vi "Command Wait.vi"(2 "Input Robot Commands":T1, 3 "Startup":bool, 4 "Cmd Parameter 4":string, 5 "Cmd Parameter 3":dbl, 6 "Cmd Parameter 2":dbl, 7 "Cmd Parameter 1":dbl) -> (0 "Output Robot Commands":T1, 1 "Completed":bool)   [LabVIEW 2016]
uses:
  Subsystems/All Robot Commands.ctl
  Subsystems/Drive and Climb SS/Drive + Climb Commands 2017.ctl
  Subsystems/Gear Delivery SS/Gear Delivery Commands.ctl
  Subsystems/Conveyor and Shooter SS/Conveyor and Shooter Commands.ctl
  Subsystems/Ball Intake SS/Ball Intake Commands.ctl
  Command Execution State.ctl
panel:
  # "Sample robot\ncontrol output.\nReplace with \nactual teleop \ncontrol signal \nstructure."
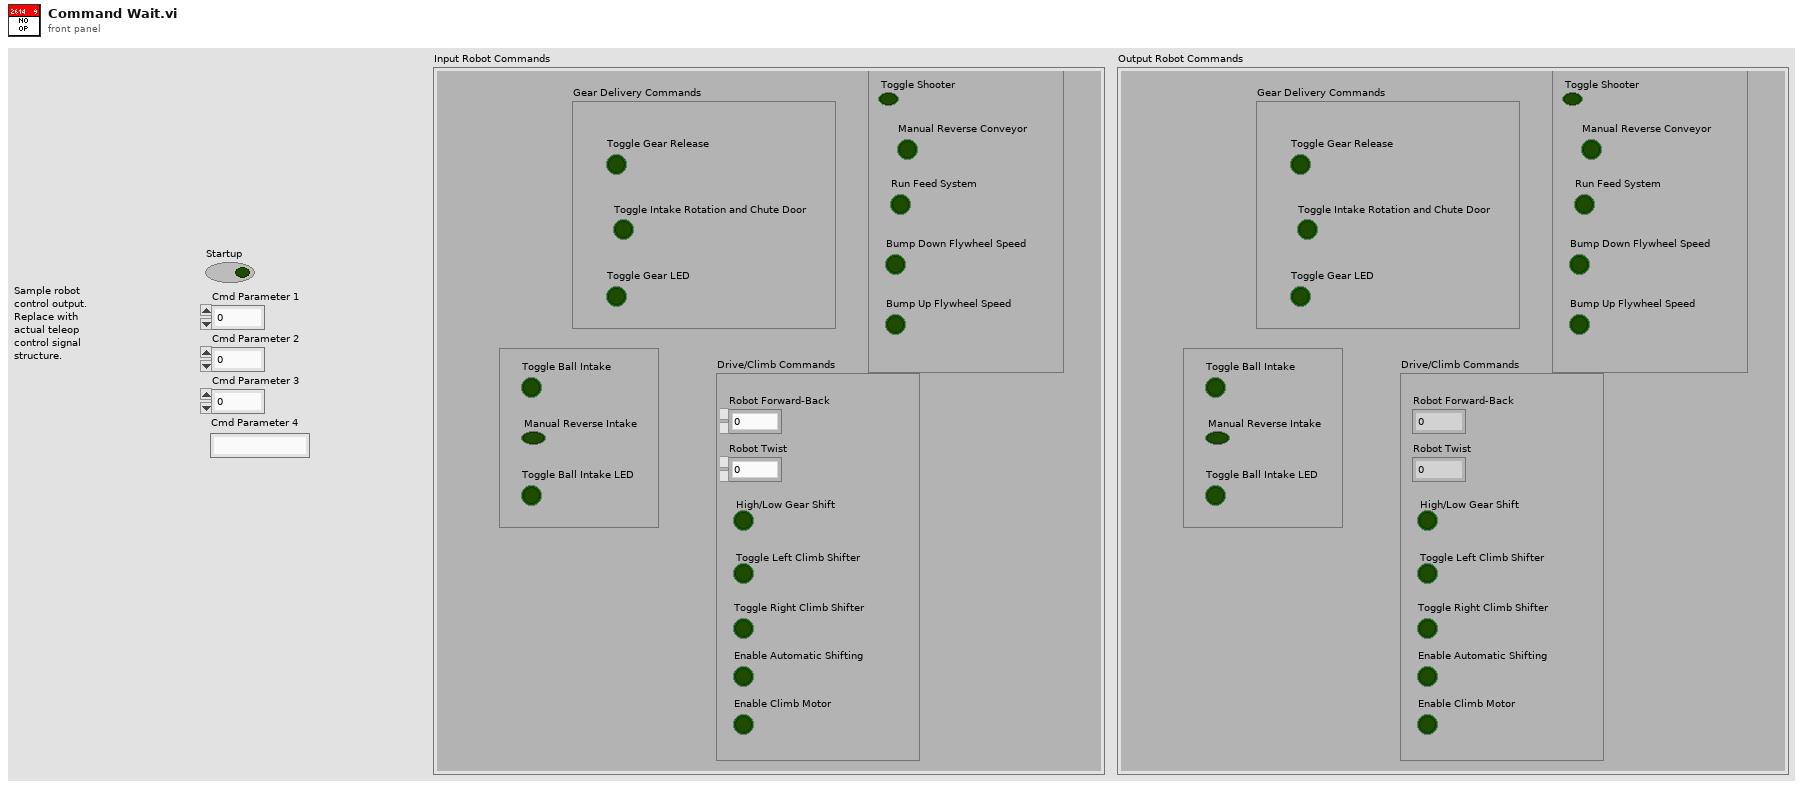
[diagram p1: front panel]
types:
  T1 = typedef "All Robot Commands.ctl" = cluster{"Drive/Climb Commands":T2, "Gear Delivery Commands":T3, "Shooter and Conveyor Commands":T4, "Ball Intake Commands":T5}
  T2 = typedef "Drive + Climb Commands 2017.ctl" = cluster{"Robot Forward-Back":dbl, "Robot Twist":dbl, "High/Low Gear Shift":bool, "Toggle Left Climb Shifter":bool, "Toggle Right Climb Shifter":bool, "Enable Automatic Shifting":bool, "Enable Climb Motor ":bool}
  T3 = typedef "Gear Delivery Commands.ctl" = cluster{"Toggle Gear Release":bool, "Toggle Intake Rotation and Chute Door":bool, "Toggle Gear LED":bool}
  T4 = typedef "Conveyor and Shooter Commands.ctl" = cluster{"Toggle Shooter":bool, "Manual Reverse Conveyor":bool, "Run Feed System":bool, "Bump Down Flywheel Speed":bool, "Bump Up Flywheel Speed":bool}
  T5 = typedef "Ball Intake Commands.ctl" = cluster{"Toggle Ball Intake":bool, "Manual Reverse Intake":bool, "Toggle Ball Intake LED":bool}
  T6 = typedef "Command Execution State.ctl" = enum16{"Initialize", "Execute", "Finish"}
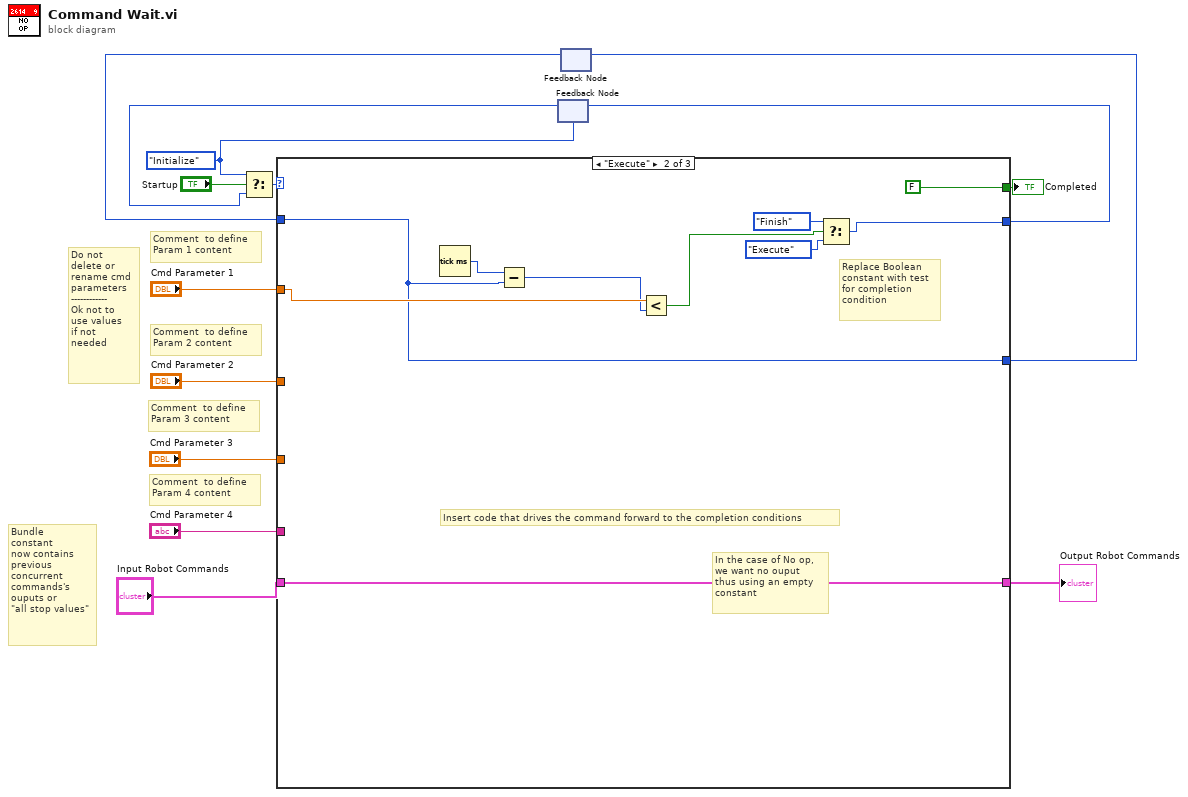
[diagram p0: block diagram]
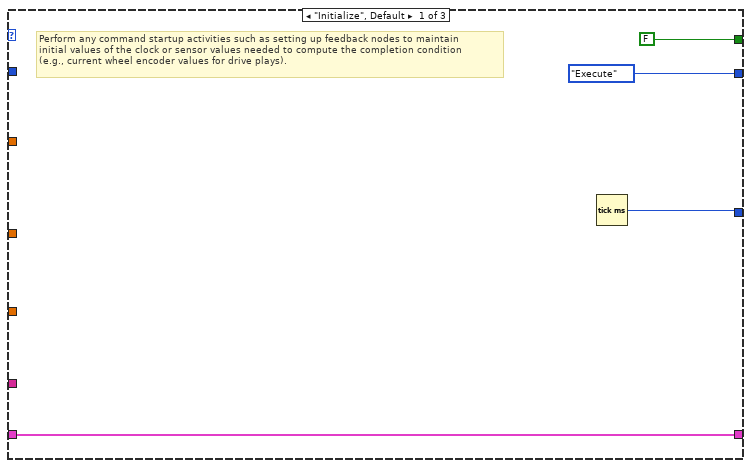
[diagram p2: hidden frame]
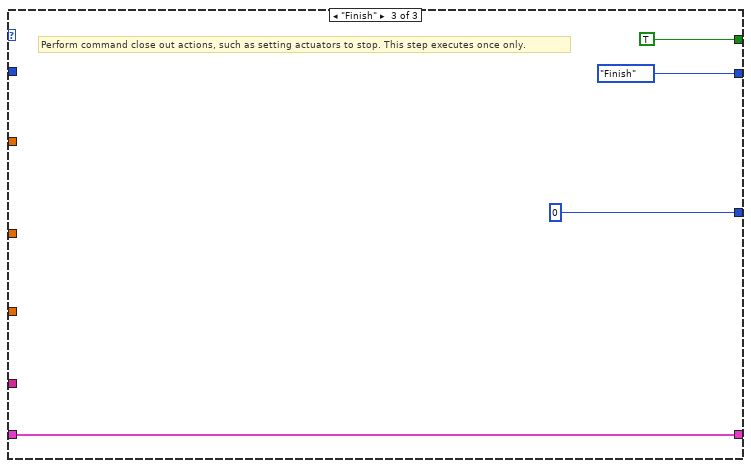
[diagram p3: hidden frame]
diagram:
  w9 = Command_Execution_State."Initialize" ("Play State")
  # "Comment  to define\nParam 4 content"
  # "Comment  to define\nParam 3 content"
  # "Bundle \nconstant\nnow contains\nprevious \nconcurrent\ncommands's\nouputs or\n\"all stop values\""
  # "Do not \ndelete or\nrename cmd\nparameters\n------------\nOk not to \nuse values\nif not \nneeded"
  # "Comment  to define\nParam 2 content"
  # "Comment  to define\nParam 1 content"
  n1 = feedback #1(w9) -> (w10:T6)
  n2 = Select(t=w9, s="Startup", f=w10) -> (s? t:f=w14:T6)
  n3 = feedback #2() -> (w1:u32)  [unwired: 1 in]
  n4 = case shown="\"Execute\"" w14 {
    tunnel: [FALSE FALSE TRUE] -> w12
    tunnel: [Command_Execution_State."Execute" ("Play State") w22 Command_Execution_State."Finish" ("f")] -> w11
    tunnel: "Cmd Parameter 1" -> [_ w26 _]
    tunnel: "Cmd Parameter 2" -> [_ _ _]
    tunnel: [w16 w27 w30] -> w5
    tunnel: "Input Robot Commands" -> [w16 w27 w30]
    tunnel: "Cmd Parameter 3" -> [_ _ _]
    tunnel: "Cmd Parameter 4" -> [_ _ _]
    tunnel: [w15 w19 0] -> w2
    tunnel: w1 -> [_ w19 _]
    frame "Initialize", Default {
      # "Perform any command startup activities such as setting up feedback nodes to maintain \ninitial values of the clock or sensor values needed to compute the completion condition\n(e.g., current wheel encoder values for drive plays)."
      n5 = Tick Count (ms)() -> (millisecond timer value=w15:u32)
    }
    frame "Execute" {
      # "In the case of No op, \nwe want no ouput \nthus using an empty \nconstant"
      # "Replace Boolean\nconstant with test \nfor completion \ncondition"
      # "Insert code that drives the command forward to the completion conditions"
      n6 = Tick Count (ms)() -> (millisecond timer value=w21:u32)
      n7 = Subtract(x=w21, y=w19) -> (x-y=w20:u32)
      n8 = Less?(x=w26, y=w20) -> (x < y?=w25:bool)
      n9 = Select(t=Command_Execution_State."Finish" ("Play State"), s=w25, f=Command_Execution_State."Execute" ("Play State")) -> (s? t:f=w22:T6)
    }
    frame "Finish" {
      # "Perform command close out actions, such as setting actuators to stop. This step executes once only."
    }
  }
  "Completed" <- w12
  "Output Robot Commands" <- w5
  n10 = feedback-in #1(w11) -> ()
  n11 = feedback-in #2(w2) -> ()
